vi "Open WebDAV Ref.vi"(8 "error in (no error)":errorcluster, 11 "IPAddress":string) -> (0 "error out":errorcluster, 1 "Password Output":string, 2 "Username Output":string, 3 "Refnum out":T1)   [LabVIEW 2014]
doc: "Attempts to connect with Admin/\"Blank\". If that fails, it prompts for a username and password"
uses:
  <vilib>/WebDAVClient/Advanced/SessionHandle.ctl
  <vilib>/WebDAVClient/NI_WebDAV.lvlib
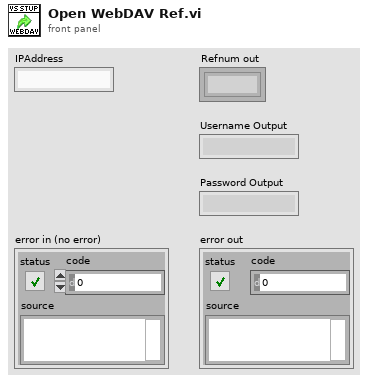
[diagram p1: front panel]
types:
  T1 = typedef "NI_WebDAV.lvlib/SessionHandle.ctl" = refnum<k1>
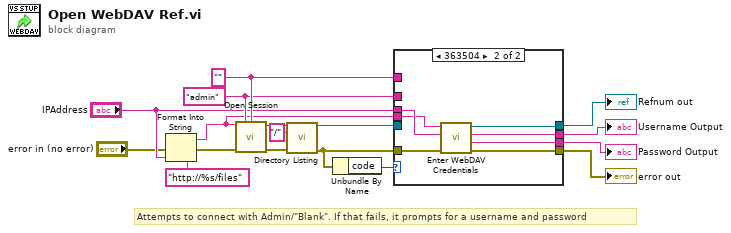
[diagram p0: block diagram]
diagram:
  w14 = "admin" ("username")
  w16 = "" ("password")
  # "Attempts to connect with Admin/\"Blank\". If that fails, it prompts for a username and password"
  n1 = Format Into String(format string="http://%s/files", error in="error in (no error)", "IPAddress") -> (resulting string=w10:string, error out=w2:errorcluster)  [unwired: 1 in]
  n2 = call <vilib>:"Open Session.vi"("host uri prefix"=w10, "username"=w14, "password"=w16, "error in (no error)"=w2) -> ("session handle out"=w4:T1, "error out"=w5:errorcluster)  [unwired: 10 in]
  n3 = call <vilib>:"Directory Listing.vi"("session handle"=w4, "relative uri"="/", "error in (no error)"=w5) -> ("session handle out"=w11:T1, "error out"=w8:errorcluster)  [unwired: 9 in, 2 out]
  n4 = Unbundle By Name(w8) -> ("code"=w7:i32)
  n5 = case shown="363504" w7 {
    tunnel: w8 -> [w21 w28]
    tunnel: [w21 w25] -> w13
    tunnel: "IPAddress" -> [_ w27]
    tunnel: w10 -> [_ w26]
    tunnel: w11 -> [w20 _]
    tunnel: [w20 w24] -> w12
    tunnel: w14 -> [w19 _]
    tunnel: [w19 w23] -> w15
    tunnel: w16 -> [w18 _]
    tunnel: [w18 w22] -> w17
    frame Default {
    }
    frame 363504 {
      n6 = call "Enter WebDAV Credentials.vi"("error in (no error)"=w28, "IP Address"=w27, "host uri prefix"=w26) -> ("error out"=w25:errorcluster, "Password Output"=w22:string, "Username Output"=w23:string, "WebDAV session handle out"=w24:T1)  [unwired: 5 in]
    }
  }
  "Password Output" <- w17
  "Username Output" <- w15
  "error out" <- w13
  "Refnum out" <- w12
